vi "IMU_Noise.vi"() -> ()   [LabVIEW 2019]
uses:
  <vilib>/numeric/Random Number (Range) I64.vi
  <vilib>/numeric/sub_Random U32.vi
  <vilib>/Analysis/NI_AALBase.lvlib
panel:
  out "Measured_IMU(degrees)":dbl
  out "Waveform Chart":dbl(graph)
  out "Gaussian noise pattern":dbl[](array[numeric])
  in  "standard deviation(for gaussian)":dbl=0.17 format="%0.2f"
  in  "True_IMU(angle)":dbl
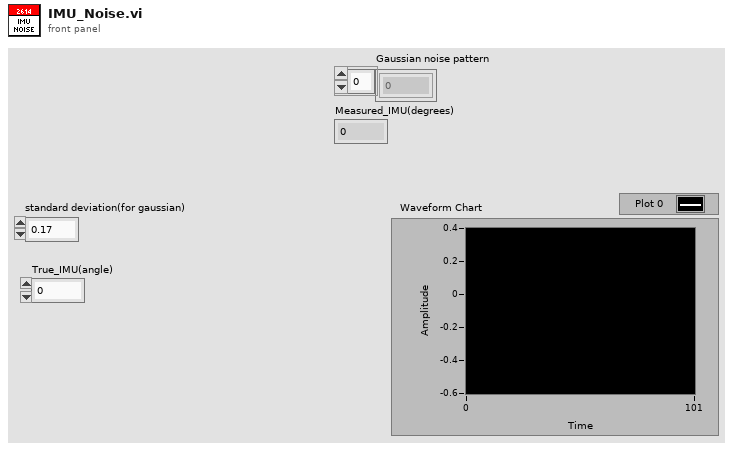
[diagram p1: front panel]
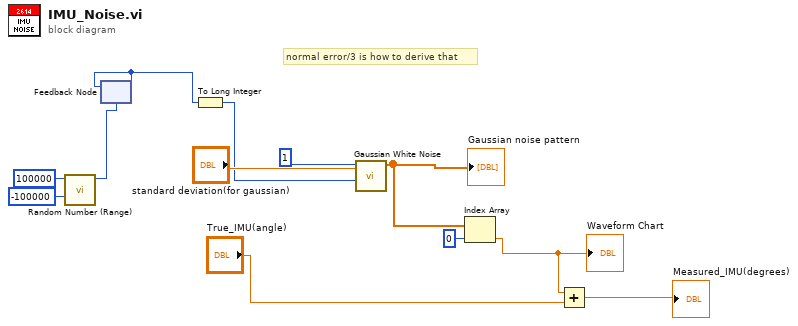
[diagram p0: block diagram]
diagram:
  # "normal error/3 is how to derive that"
  n1 = call-poly <vilib>:"Random Number (Range).vi"("lower bound (-100)"=i64 -100000, "upper bound (100)"=i64 100000) -> ("number"=w6:i64)  [unwired: 9 in]
  n2 = feedback #1(w6) -> (w3:i64)
  n3 = feedback-in #1(w3) -> ()
  n4 = To Long Integer(number=w3) -> (32bit integer=w2:i32)
  n5 = call <vilib>:"Gaussian White Noise.vi"("seed"=w2, "standard deviation"="standard deviation(for gaussian)", "samples"=1) -> ("Gaussian noise pattern"=w10:dbl[])  [unwired: 7 in, 1 out]
  "Gaussian noise pattern" <- w10
  n6 = Index Array(array=w10, index=0) -> (element=w8:dbl)
  "Waveform Chart" <- w8
  n7 = Add(x=w8, y="True_IMU(angle)") -> (x+y=→"Measured_IMU(degrees)":dbl)
